vi "CRCTest.vi"(10 "unsigned byte array":u8[](array[numeric])) -> (1 "size(s)":i32, 2 "length":i32)   [LabVIEW 2017]
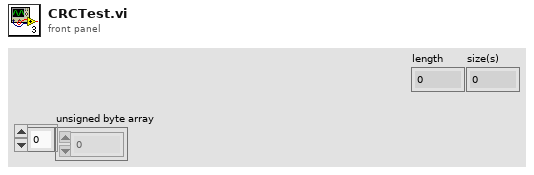
[diagram p1: front panel]
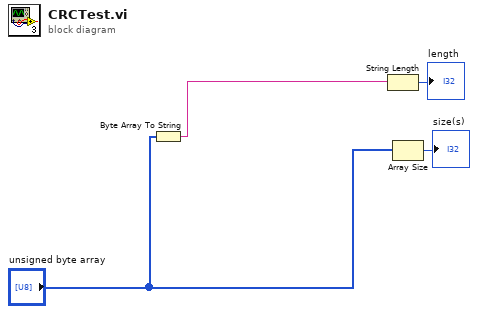
[diagram p0: block diagram]
diagram:
  n1 = Byte Array To String(unsigned byte array="unsigned byte array") -> (string=w1:string)
  n2 = String Length(string=w1) -> (length=→"length":i32)
  n3 = Array Size(array="unsigned byte array") -> (size(s)=→"size(s)":i32)
